vi "Anything_To_Variant.vi"(8 "error in (no error)":errorcluster, 10 "Options":T1, 11 "Anything":variant) -> (0 "error out":errorcluster, 3 "Serialized Variant":variant)   [LabVIEW 2020, in "BlueSerialization.lvlib" / "BlueSerializer.lvclass"]
uses:
  BlueSerializer.lvclass
  SerializeOptionsPayload.ctl
  SerializeOptions.ctl
  ClassNameCacheMap.ctl
  ClassNameObj.ctl
  BlueSerializable/BlueSerializable.lvclass
  SerializeSliceCalc.vi
  BlueSerializable/GetSerializableData_StaticCommunity.vi
  SerializeBuildHeader.vi
  GetClassNameArray.vi
  SerializeSliceCalcString.vi
  BlueSerializable/SetSerializeSliceClass_StaticCommunity.vi
  GetClassNameAndVersion.vi
  GetParentClassesHiererchy.vi
  ClassNameCacheWrite.vi
  LVOOP Get Default Object Inline.vi
  GetLastCompatibleVersion.vi
  <vilib>/Utility/LVClass/Get LV Class Default Value By Name.vi
  <vilib>/Utility/EditLVLibs/LVClass/Get Mutation History.vi
  <vilib>/Utility/error.llb/Error Cluster From Error Code.vi
  <vilib>/ErrorRing/Error Ring.xnode
  BlueSerializer.lvclass/BlueSerializer.ctl
  <vilib>/Utility/Data Type/NI_Data Type.lvlib
  <vilib>/JDP Science/JDP Science Common Utilities/JDP Utility.lvlib
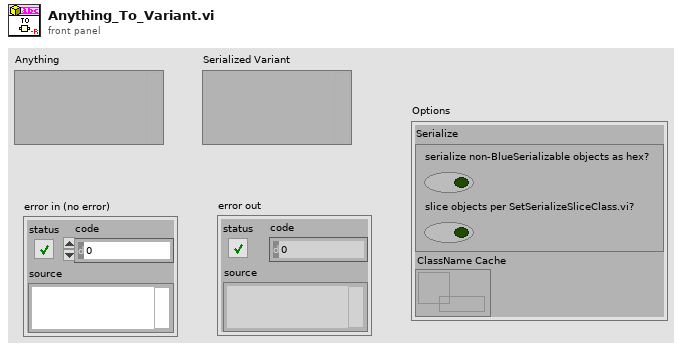
[diagram p1: front panel]
types:
  T1 = typedef "BlueSerialization.lvlib/BlueSerializer.lvclass/SerializeOptionsPayload.ctl" = cluster{"Serialize":T2, "ClassName Cache":refnum<data-value>}
  T2 = typedef "BlueSerialization.lvlib/BlueSerializer.lvclass/SerializeOptions.ctl" = cluster{"serialize non-BlueSerializable objects as hex?":bool, "slice objects per SetSerializeSliceClass.vi?":bool}
  T3 = typedef "NI_Data Type.lvlib/Data Type.ctl" = enum8{"Invalid Type", "Void", "I8", "I16", "I32", "I64", "U8", "U16", "U32", "U64", "Single Float", "Double Float", "Extended Float", "Single Complex", "Double Complex", "Extended Complex", "Enum U8", "Enum U16", "Enum U32", "Enum U64", "Single Float With Unit", "Double Float With Unit", "Extended Float With Unit", "Single Complex with Unit", "Double Complex with Unit", "Extended Complex with Unit", "Boolean", "String", "Path", "Picture", "Tag", "Array", "Cluster", "Variant", "LV Variant", "Waveform", "Timestamp", "Digital Waveform", "Digital Data", "ExpressData", "Refnum", "External Data", "VI", "Poly VI", "LabVIEW Class Instance", "Fixed Point", "Set Collection", "Map Collection"}
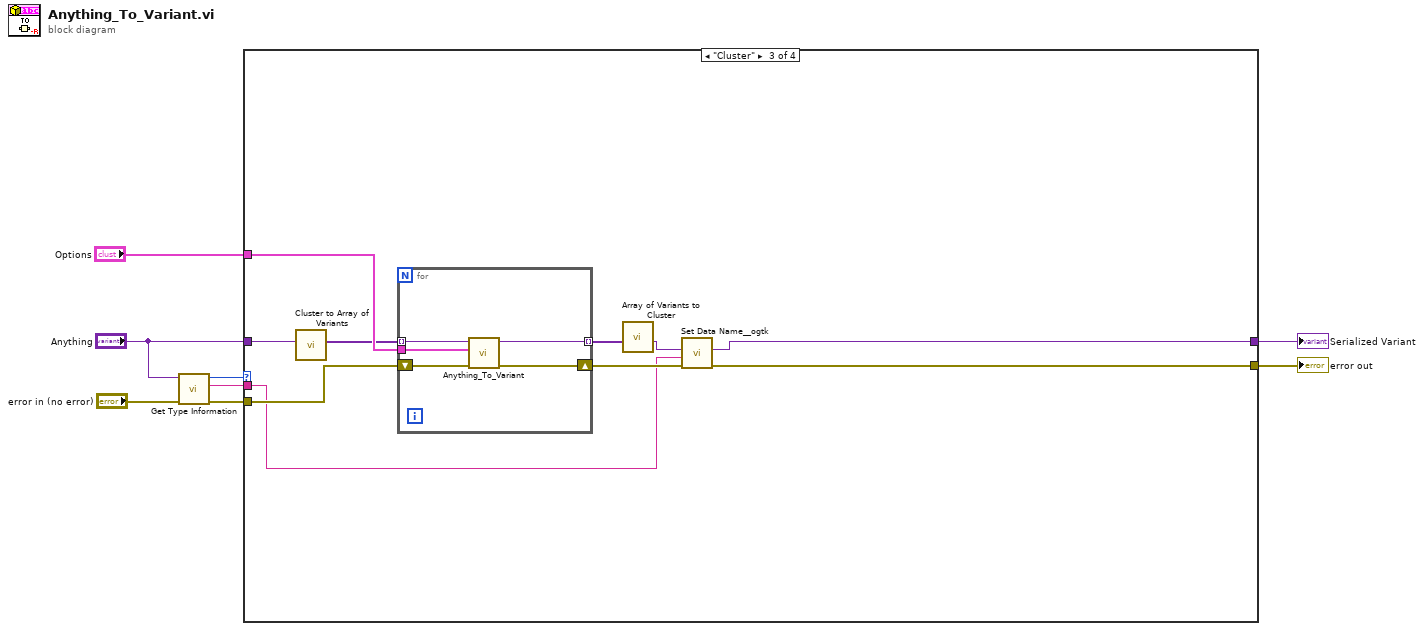
[diagram p0: block diagram]
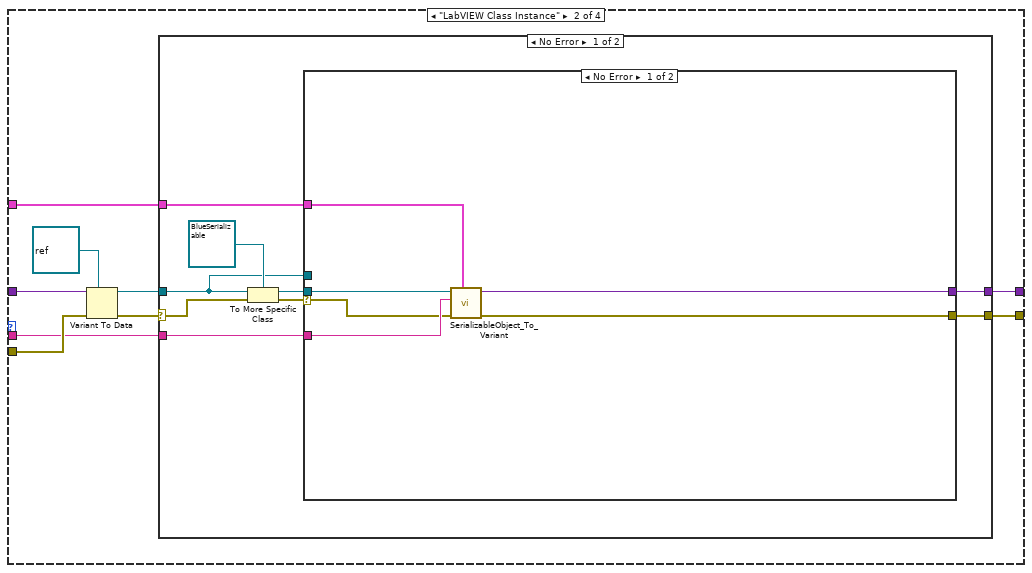
[diagram p3: hidden frame]
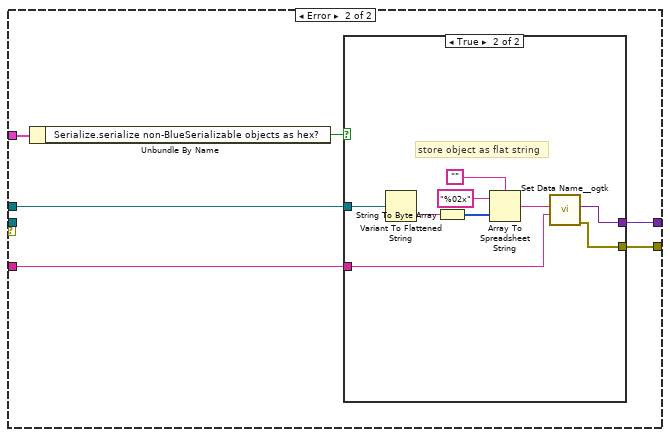
[diagram p4: hidden frame]
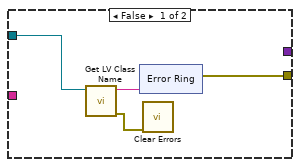
[diagram p5: hidden frame]
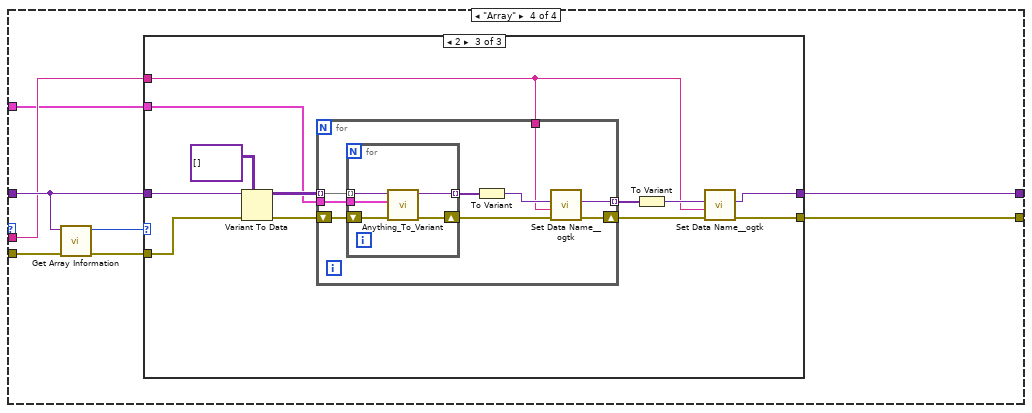
[diagram p7: hidden frame]
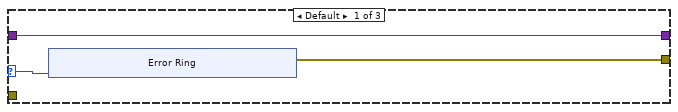
[diagram p8: hidden frame]
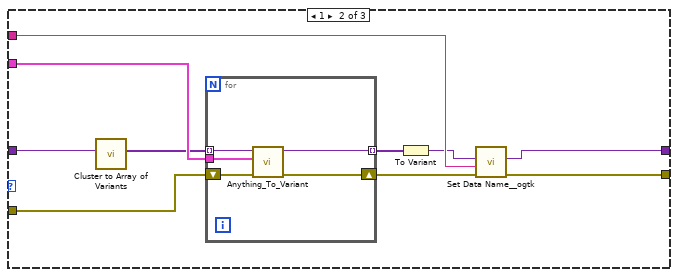
[diagram p9: hidden frame]
diagram:
  n1 = call <vilib>:"Get Type Information.vi"("error in (no error)"="error in (no error)", "variant"="Anything") -> ("error out"=w4:errorcluster, "name"=w2:string, "type"=w7:T3)  [unwired: 5 in, 2 out]
  n2 = case shown="\"Cluster\"" w7 {
    tunnel: "Anything" -> [w9 w19 w70 w81]
    tunnel: [w9 w17 w63 w80] -> w5
    tunnel: w4 -> [w10 w18 w68 w84]
    tunnel: [w10 w16 w62 w79] -> w3
    tunnel: w2 -> [_ w15 w64 w78]
    tunnel: "Options" -> [_ w11 w71 w77]
    frame Default {
    }
    frame "LabVIEW Class Instance" {
      n3 = Variant To Data(error in=w18, type=refnum<class> refnum ("LabVIEW Object"), Variant=w19) -> (data=w12:refnum<class>, error out=w13:errorcluster)
      n4 = case shown="No Error" w13 {
        selector: w13 -> [w23 w61]
        tunnel: [w28 _] -> w17
        tunnel: [w27 w61] -> w16
        tunnel: w15 -> [w26 _]
        tunnel: w12 -> [w21 _]
        tunnel: w11 -> [w20 _]
        frame No Error {
          n5 = To More Specific Class(target class=refnum<class "BlueSerializable.lvclass"> refnum ("Class to Serialize"), reference=w21, error in=w23) -> (specific class reference=w24:refnum<class "BlueSerializable.lvclass">, error out=w22:errorcluster)
          n6 = case shown="No Error" w22 {
            selector: w22 -> [w30 _]
            tunnel: [w34 w36] -> w28
            tunnel: [w33 w39] -> w27
            tunnel: w26 -> [w32 w35]
            tunnel: w24 -> [w31 _]
            tunnel: w21 -> [_ w40]
            tunnel: w20 -> [w29 w38]
            frame No Error {
              n7 = call "SerializableObject_To_Variant.vi"("Options"=w29, "error IO"=w30, "Object Name"=w32, "Class to Serialize"=w31) -> ("error out"=w33:errorcluster, "Vcluster"=w34:variant)  [unwired: 6 in]
            }
            frame Error {
              n8 = Unbundle By Name(w38) -> ("Serialize.serialize non-BlueSerializable objects as hex?"=w37:bool)
              n9 = case shown="True" w37 {
                tunnel: w40 -> [w44 w56]
                tunnel: [w43 w52] -> w39
                tunnel: [_ w53] -> w36
                tunnel: w35 -> [_ w54]
                frame False {
                  n10 = call <vilib>:"Get LV Class Name.vi"("object"=w44) -> ("error out"=w41:errorcluster, "class name"=w42:string)  [unwired: 9 in]
                  n11 = xnode "Error Ring"("parameter 0"=w42) -> ("error out"=w43:errorcluster)
                  n12 = call <vilib>:"Clear Errors.vi"("error in (no error)"=w41) -> ()  [unwired: 5 in, 2 out]
                }
                frame True {
                  # "store object as flat string"
                  n13 = Variant To Flattened String(Variant=w56) -> (data string=w60:string)  [unwired: 1 out]
                  n14 = String To Byte Array(string=w60) -> (unsigned byte array=w59:u8[])
                  n15 = Array To Spreadsheet String(delimiter (Tab)="", array=w59, 3:"%02x" ("format string")) -> (spreadsheet string=w55:string)
                  n16 = call <userlib>:"Set Data Name__ogtk.vi"("Data Name"=w54, "Data"=w55) -> ("error out"=w52:errorcluster, "Renamed Data"=w53:variant)  [unwired: 8 in]
                }
              }
            }
          }
        }
        frame Error {
        }
      }
    }
    frame "Cluster" {
      n17 = call <vilib>:"Cluster to Array of Variants.vi"("Cluster"=w70) -> ("Array of Cluster Elements"=w69:variant[])  [unwired: 10 in]
      n18 = for {
        tunnel: w69 -> [w76] mode=indexing
        tunnel: [w75] -> w67 mode=indexing
        shift-right: [w73] -> w66
        shift-left: w68 -> [w74]
        tunnel: w71 -> [w72]
        n19 = call "Anything_To_Variant.vi"("error in (no error)"=w74, "Options"=w72, "Anything"=w76) -> ("error out"=w73:errorcluster, "Serialized Variant"=w75:variant)  [unwired: 7 in]
      }
      n20 = call <vilib>:"Array of Variants to Cluster.vi"("Array of Variants"=w67) -> ("Cluster of Variants"=w65:variant)  [unwired: 10 in]
      n21 = call <userlib>:"Set Data Name__ogtk.vi"("error in (no error)"=w66, "Data Name"=w64, "Data"=w65) -> ("error out"=w62:errorcluster, "Renamed Data"=w63:variant)  [unwired: 7 in]
    }
    frame "Array" {
      n22 = call <vilib>:"Get Array Information.vi"("error in (no error)"=w84, "variant"=w81) -> ("error out"=w82:errorcluster, "number of dimensions"=w83:i32)  [unwired: 6 in, 2 out]
      n23 = case shown="2" w83 {
        selector: w83 -> [w86 _ _]
        tunnel: w82 -> [_ w101 w119]
        tunnel: w81 -> [w87 w103 w120]
        tunnel: [w87 w96 w112] -> w80
        tunnel: [w85 w95 w111] -> w79
        tunnel: w78 -> [_ w99 w110]
        tunnel: w77 -> [_ w104 w116]
        frame Default {
          n24 = xnode "Error Ring"("parameter 0"=w86) -> ("error out"=w85:errorcluster)
        }
        frame 1 {
          n25 = call <vilib>:"Cluster to Array of Variants.vi"("Cluster"=w103) -> ("Array of Cluster Elements"=w102:variant[])  [unwired: 10 in]
          n26 = for {
            tunnel: w102 -> [w109] mode=indexing
            tunnel: [w108] -> w100 mode=indexing
            shift-right: [w106] -> w98
            shift-left: w101 -> [w107]
            tunnel: w104 -> [w105]
            n27 = call "Anything_To_Variant.vi"("error in (no error)"=w107, "Options"=w105, "Anything"=w109) -> ("error out"=w106:errorcluster, "Serialized Variant"=w108:variant)  [unwired: 7 in]
          }
          n28 = To Variant(anything=w100) -> (Variant=w97:variant)
          n29 = call <userlib>:"Set Data Name__ogtk.vi"("error in (no error)"=w98, "Data Name"=w99, "Data"=w97) -> ("error out"=w95:errorcluster, "Renamed Data"=w96:variant)  [unwired: 7 in]
        }
        frame 2 {
          n30 = Variant To Data(error in=w119, type=variant[][] [], Variant=w120) -> (data=w118:variant[][], error out=w117:errorcluster)
          n31 = for {
            tunnel: w118 -> [w130] mode=indexing
            shift-right: [w123] -> w115
            shift-left: w117 -> [w129]
            tunnel: w110 -> [w124]
            tunnel: w116 -> [w128]
            tunnel: [w122] -> w114 mode=indexing
            n32 = for {
              tunnel: w130 -> [w135] mode=indexing
              tunnel: [w134] -> w126 mode=indexing
              shift-right: [w132] -> w125
              shift-left: w129 -> [w133]
              tunnel: w128 -> [w131]
              n33 = call "Anything_To_Variant.vi"("error in (no error)"=w133, "Options"=w131, "Anything"=w135) -> ("error out"=w132:errorcluster, "Serialized Variant"=w134:variant)  [unwired: 7 in]
            }
            n34 = To Variant(anything=w126) -> (Variant=w127:variant)
            n35 = call <userlib>:"Set Data Name__ogtk.vi"("error in (no error)"=w125, "Data Name"=w124, "Data"=w127) -> ("error out"=w123:errorcluster, "Renamed Data"=w122:variant)  [unwired: 7 in]
          }
          n36 = To Variant(anything=w114) -> (Variant=w113:variant)
          n37 = call <userlib>:"Set Data Name__ogtk.vi"("error in (no error)"=w115, "Data Name"=w110, "Data"=w113) -> ("error out"=w111:errorcluster, "Renamed Data"=w112:variant)  [unwired: 7 in]
        }
      }
    }
  }
  "error out" <- w3
  "Serialized Variant" <- w5
